vi "Read Dev Format.vi"(8 "error in (no error)":errorcluster, 11 "VISA resource name":refnum<visa-resource-name>) -> (0 "error out":errorcluster, 2 "dev format":T1, 3 "VISA resource name out":refnum<visa-resource-name>)   [LabVIEW 2019, in "Andeen-Hagerling 2700A.lvlib"]
doc: "Returns the deviation format applied to deviation results.\n\n0 - Deviation measurement results are\n reported in absolute pF and jpF units. A\n measurement at the Deviation Setpoint will\n be reported as DPointC pF and DPointL\n jpF.\n1 - Deviation measurement results are\n reported as simple differences from the\n Deviation Setpoint in units of pF and jpF.\n A measurement at the Deviation Setpoint\n will be reported as 0 pF and 0 jpF.\n2 Deviation measurement results are\n reported as differences from the Deviation\n Setpoint as a percentage of the Deviation\n Setpoint. A measurement at the Deviation\n Setpoint will be reported as 0% for both\n capacitance and loss.\n3 Deviation measurement results are\n reported as differences from the Deviation\n Setpoint as a percentage of the deviation\n input span. Measurement values at the\n DBndLo and DBndUp bounds will be\n reported as -50% and +50% respectively.\n4 Deviation measurement results are\n reported as differences from the Deviation\n Setpoint as a percentage of the deviation\n input span. Measurement values at the\n DBndLo and DBndUp bounds will be\n reported as -100% and +100% respectively."
uses:
  Andeen-Hagerling 2700A.lvlib
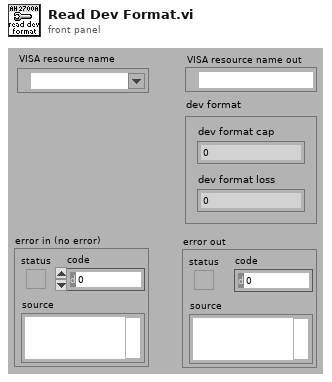
[diagram p1: front panel]
types:
  T1 = cluster{"dev format cap":i32, "dev format loss":i32}
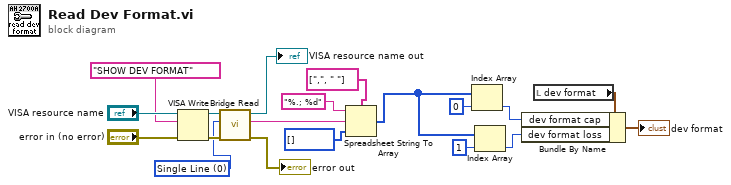
[diagram p0: block diagram]
diagram:
  w1 = u16 0 items=["Single Line", "Multi-Line"] ("Multiline")
  n1 = VISA Write(VISA resource name="VISA resource name", write buffer="SHOW DEV FORMAT" ("command"), error in (no error)="error in (no error)") -> (VISA resource name out=w6:refnum<visa-resource-name>, error out=w5:errorcluster)  [unwired: 1 out]
  n2 = call "Bridge Read.vi"("error in (no error)"=w5, "multiline"=w1, "VISA resource name"=w6) -> ("error out"=→"error out":errorcluster, "read buffer"=w2:string, "VISA resource name out"=→"VISA resource name out":refnum<visa-resource-name>)  [unwired: 6 in]
  n3 = Spreadsheet String To Array(delimiter (Tab)=string[] [",", " "], format string="%.; %d", spreadsheet string=w2, array type (2D Dbl)=i32[] []) -> (array=w12:i32[])
  n4 = Index Array(array=w12, index=0) -> (element=w9:i32)
  n5 = Index Array(array=w12, index=1) -> (element=w8:i32)
  n6 = local read "dev format"() -> (w10:T1)
  n7 = Bundle By Name(cluster=w10, "dev format cap"=w9, "dev format loss"=w8) -> (→"dev format":T1)
